vi "Update Aisle of Records.vi"(0 "GUI Aisle In":T1[](array[typedef]) {"Night Cycle Count" format="%04d"; "Dryer Details"."Stop Dryer" items=["NO", "YES"]; "Dryer Details"."24 Hour Water Injection" items=["NO", "YES"]; "Dryer Details"."Run w/o Newfi" items=["NO", "YES"]; "Day Cycle Count" format="%04d"}, 1 "Day Shift?":bool, 7 "Dryer Com Info":T3[](array[typedef]), 9 "Current Agilent Data":dbl[](array[numeric]), 11 "Agilent Station Data Index Array":i32[][](array[numeric])) -> (4 "Aisle Array Out":T1[](array[typedef]) {"Night Cycle Count" format="%04d"; "Dryer Details"."Stop Dryer" items=["NO", "YES"]; "Dryer Details"."24 Hour Water Injection" items=["NO", "YES"]; "Dryer Details"."Run w/o Newfi" items=["NO", "YES"]; "Day Cycle Count" format="%04d"})   [LabVIEW 2012]
uses:
  Dryer.ctl
  Dryer Details.ctl
  Dryer Com Port Info.ctl
  Dryer Status Ctrl.ctl
  Update Wilt GUI Control.ctl
panel:
  # "D"
  # "N"
  # "D"
  # "N"
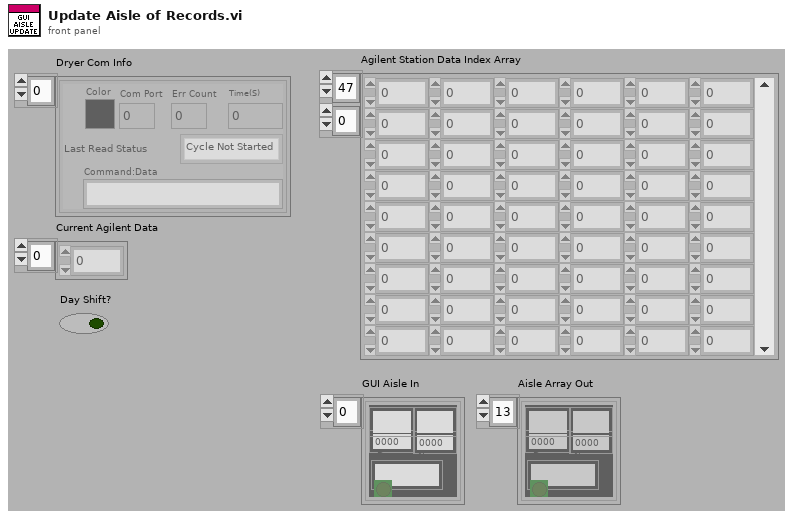
[diagram p1: front panel]
types:
  T1 = typedef "Dryer.ctl" = cluster{"Lab ID":string, "Day Cycle Count":i32, "Station Label":string, "Dryer Details":T2, "Sample Record ":string[], "Hist Record ":string[][], "Status Color":u32, "Boolean":bool, "Com Port":u8, "Bad Com Count":i32, "Current Run Start Time":dbl, "Night Cycle Count":i32, "Station Index":i32, "Cycle Index":string, "Audit Alert":bool}
  T2 = typedef "Dryer Details.ctl" = cluster{"Station":string, "Cycle Count Day":string, "Status":string, "Debug ASCII":string, "Notes":string, "Lab ID":string, "Total Time On":string, "TR Number":string, "Cycle Count Night":string, "Time On Day":string, "Time On Night":string, "Run w/o Newfi":i32, "24 Hour Water Injection":i32, "Stop Dryer":i32}
  T3 = typedef "Dryer Com Port Info.ctl" = cluster{"Color":u32, "Last Read Status":T4, "Command:Data":string, "Com Port":u8, "Time(S)":dbl, "Err Count":u32}
  T4 = typedef "Dryer Status Ctrl.ctl" = enum16{"Cycle Not Started", "Cycle Running", "Paused", "Cycle Completed", "Eval Mode Entered", "Err", "Pause (No GEA2)"}
  T5 = typedef "Update Wilt GUI Control.ctl" = enum16{"Init Station Number", "Update Detail Data", "Update Status", "Init Com Port Num", "Update Sample Info", "Reset All Cycles"}
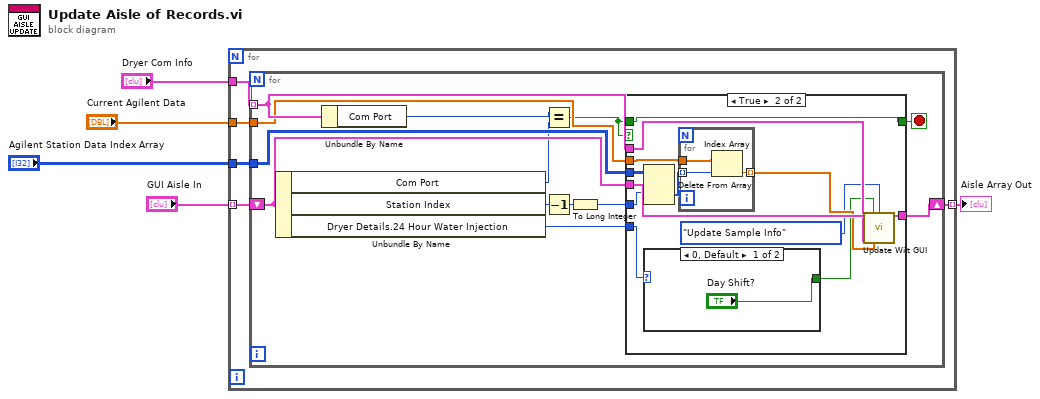
[diagram p0: block diagram]
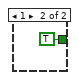
[diagram p3: hidden frame]
diagram:
  n1 = for {
    tunnel: "GUI Aisle In" -> [w10] mode=indexing
    tunnel: "Dryer Com Info" -> [w9]
    tunnel: [w8] -> w5 mode=indexing
    tunnel: "Agilent Station Data Index Array" -> [w7]
    tunnel: "Current Agilent Data" -> [w6]
    n2 = for {
      tunnel: w9 -> [w20] mode=indexing
      shift-right: [w21] -> w8
      shift-left: w10 -> [w22]
      tunnel: w7 -> [w19]
      tunnel: w6 -> [w17]
      stop <- w16 stop-if-true
      n3 = Unbundle By Name(w22) -> ("Com Port"=w18:u8, "Station Index"=w13:i32, "Dryer Details.24 Hour Water Injection"=w11:i32)
      n4 = Unbundle By Name(w20) -> ("Com Port"=w23:u8)
      n5 = Equal?(x=w23, y=w18) -> (x = y?=w15:bool)
      n6 = Decrement(x=w13) -> (x-1=w14:i32)
      n7 = To Long Integer(number=w14) -> (32bit integer=w12:i32)
      n8 = case shown="True" w15 {
        tunnel: w22 -> [w25 w37]
        tunnel: w20 -> [_ w35]
        tunnel: [w25 w36] -> w21
        tunnel: w19 -> [_ w34]
        tunnel: w12 -> [_ w33]
        tunnel: w17 -> [_ w32]
        tunnel: [w24 w28] -> w16
        tunnel: w15 -> [w24 w28]
        tunnel: w11 -> [_ w26]
        frame False {
        }
        frame True {
          n9 = Delete From Array(array=w34, index (row)=w33) -> (deleted portion=w31:i32[])  [unwired: 2 in, 1 out]
          n10 = case shown="0, Default" w26 {
            tunnel: ["Day Shift?" TRUE ("Day Shift?")] -> w27
            frame 0, Default {
            }
            frame 1 {
            }
          }
          n11 = for {
            tunnel: w32 -> [w42]
            tunnel: w31 -> [w41] mode=indexing
            tunnel: [w40] -> w30 mode=indexing
            n12 = Index Array(array=w42, index=w41) -> (element=w40:dbl)
          }
          n13 = call "Update Wilt GUI.vi"("Dryer In"=w37, "Day Shift?"=w27, "Enum"=Update_Wilt_GUI_Control."Update Sample Info", "Dryer Status Serial Data In"=w35, "Agilent Data In"=w30) -> ("Dryer Out 2"=w36:T1)  [unwired: 8 in, 2 out]
        }
      }
    }
  }
  "Aisle Array Out" <- w5
